vi "Write as Byte Stream.vi"(6 "Offset":i32, 8 "error in (no error)":errorcluster, 9 "Byte Stream in":u8[](array[numeric]), 10 "Symbol Name":string, 11 "TwinCAT ADS in":refnum<class "TwinCAT ADS.lvclass">) -> (0 "error out":errorcluster, 1 "Byte Stream out":u8[](array[numeric]), 3 "TwinCAT ADS out":refnum<class "TwinCAT ADS.lvclass">)   [LabVIEW 2018, in "TwinCAT ADS.lvclass"]
uses:
  TwinCAT ADS.lvclass
  TwinCAT ADS.lvclass/TwinCAT ADS.ctl
  TwinCAT.Ads
  Get From Symbol Map.vi
  Get From Symbol Map Daemon.vi
  Get Symbol Map.vi
  Format String.vi
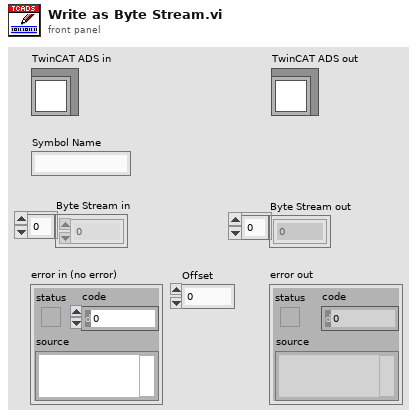
[diagram p1: front panel]
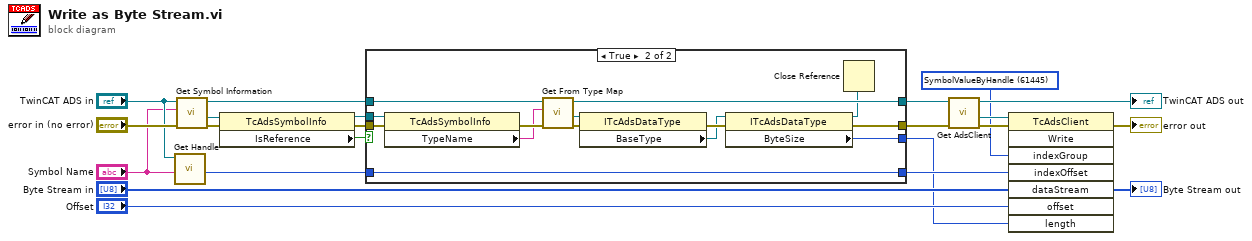
[diagram p0: block diagram]
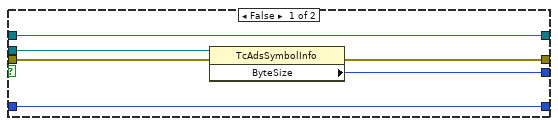
[diagram p2: hidden frame]
diagram:
  w17 = u32 61445 items=["PlcRWIB"=16384, "PlcRWOB"=16400, "PlcRWMB"=16416, "PlcRWRB"=16432, "PlcRWDB"=16448, "SymbolTable"=61440, "SymbolName"=61441, "SymbolValue"=61442, "SymbolHandleByName"=61443, "SymbolValueByName"=61444, "SymbolValueByHandle"=61445, "SymbolReleaseHandle"=61446, "SymbolInfoByName"=61447, "SymbolVersion"=61448, "SymbolInfoByNameEx"=61449, "SymbolDownload"=61450, "SymbolUpload"=61451, "SymbolUploadInfo"=61452, "SymbolNote"=61456, "IOImageRWIB"=61472, "IOImageRWIX"=61473, "IOImageRWOB"=61488, "IOImageRWOX"=61489, "IOImageClearI"=61504, "IOImageClearO"=61520, "SumCommandRead"=61568, "SumCommandWrite"=61569, "SumCommandReadWrite"=61570, "SumCommandReadEx"=61571, "SumCommandReadEx2"=61572, "SumCommandAddDevNote"=61573, "SumCommandDelDevNote"=61574, "DeviceData"=61696] ("SumCommandRead")
  n1 = call "Get Handle.vi"("Symbol Name"="Symbol Name", "TwinCAT ADS in"="TwinCAT ADS in") -> ("Handle"=w10:i32)  [unwired: 7 in, 2 out]
  n2 = call "Get Symbol Information.vi"("error in (no error)"="error in (no error)", "Symbol Name"="Symbol Name", "TwinCAT ADS in"="TwinCAT ADS in") -> ("error out"=w16:errorcluster, ".NET Symbol Information"=w15:refnum<k24>, "TwinCAT ADS out"=w14:refnum<class "TwinCAT ADS.lvclass">)  [unwired: 6 in]
  n3 = property class="TcAdsSymbolInfo"(reference=w15, error in=w16) -> (reference out=w12:refnum<k24>, error out=w13:errorcluster, "IsReference"=w11:bool)
  n4 = case shown="True" w11 {
    tunnel: w13 -> [w28 w32]
    tunnel: [w24 w40] -> w5
    tunnel: [w25 w37] -> w1
    tunnel: [w26 w35] -> w9
    tunnel: w12 -> [w27 w31]
    tunnel: w14 -> [w24 w34]
    tunnel: w10 -> [w23 w33]
    tunnel: [w23 w33] -> w6
    frame False {
      n5 = property class="TcAdsSymbolInfo"(reference=w27, error in=w28) -> (error out=w26:errorcluster, "ByteSize"=w25:i32)  [unwired: 1 out]
    }
    frame True {
      n6 = property class="TcAdsSymbolInfo"(reference=w31, error in=w32) -> (error out=w30:errorcluster, "TypeName"=w29:string)  [unwired: 1 out]
      n7 = call "Get From Type Map.vi"("error in (no error)"=w30, "Type Name"=w29, "TwinCAT ADS in"=w34) -> ("error out"=w42:errorcluster, ".NET AdsDataType"=w41:refnum<k24>, "TwinCAT ADS out"=w40:refnum<class "TwinCAT ADS.lvclass">)  [unwired: 6 in]
      n8 = property class="ITcAdsDataType"(reference=w41, error in=w42) -> (error out=w39:errorcluster, "BaseType"=w38:refnum<k24>)  [unwired: 1 out]
      n9 = property class="ITcAdsDataType"(reference=w38, error in=w39) -> (reference out=w36:refnum<k24>, error out=w35:errorcluster, "ByteSize"=w37:i32)
      n10 = Close Reference(reference=w36) -> ()  [unwired: 1 in, 1 out]
    }
  }
  n11 = call "Get AdsClient.vi"("error in (no error)"=w9, "TwinCAT ADS in"=w5) -> ("error out"=w22:errorcluster, ".NET TcAdsClient"=w21:refnum<k24>, "TwinCAT ADS out"=→"TwinCAT ADS out":refnum<class "TwinCAT ADS.lvclass">)  [unwired: 7 in]
  n12 = invoke class="TcAdsClient" method="Write"(reference=w21, error in=w22, "indexGroup"=w17, "indexOffset"=w6, "dataStream"="Byte Stream in", "offset"="Offset", "length"=w1) -> (error out=→"error out":errorcluster, "dataStream"=→"Byte Stream out":u8[])  [unwired: 1 in, 6 out]
